vi "find_note.vi"(11 "Data":waveform(dbl)[](array[waveform])) -> (2 "Note":string, 3 "Frequency":dbl[](array[numeric]))   [LabVIEW 2022 SP3]
uses:
  <vilib>/measure/NI_MAPro.lvlib
  <vilib>/measure/matone.llb/Extract Single Tone Information N Chan.vi
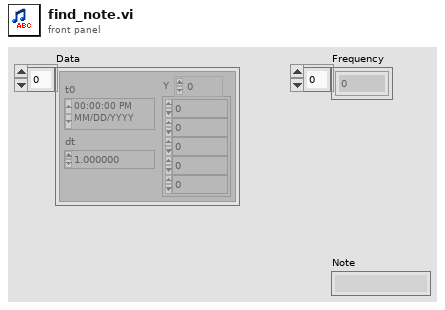
[diagram p1: front panel]
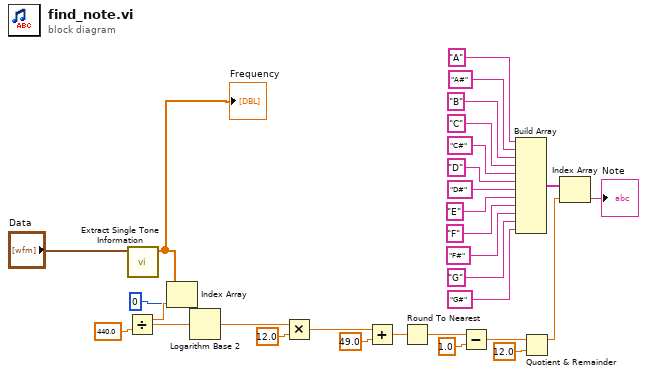
[diagram p0: block diagram]
diagram:
  n1 = call-poly <vilib>:"Extract Single Tone Information.vi"("time signals in"="Data") -> ("detected frequencies"=w26:dbl[])  [unwired: 5 in, 5 out]
  "Frequency" <- w26
  n2 = Index Array(array=w26, index=0) -> (element=w28:dbl)
  n3 = Divide(x=w28, y=440.0 ("detected frequency")) -> (x/y=w14:dbl)
  n4 = Logarithm Base 2(1:w14) -> (0:w15:dbl)
  n5 = Multiply(x=w15, y=12.0 ("detected frequency")) -> (x*y=w17:dbl)
  n6 = Add(x=w17, y=49.0 ("detected frequency")) -> (x+y=w19:dbl)
  n7 = Round To Nearest(number=w19) -> (nearest integer value=w20:dbl)
  n8 = Subtract(x=w20, y=1.0 ("detected frequency")) -> (x-y=w22:dbl)
  n9 = Build Array("A", "A#" ("element"), "B" ("element"), "C" ("element"), "C#" ("element"), "D" ("element"), "D#" ("element"), "E" ("element"), "F" ("element"), "F#" ("element"), "G" ("element"), "G#" ("element")) -> (w24:string[])
  n10 = Quotient & Remainder(x=w22, y=12.0 ("detected frequency")) -> (x-y*floor(x/y)=w25:dbl)  [unwired: 1 out]
  n11 = Index Array(array=w24, index=w25) -> (element=→"Note":string)
